vi "SteeringControl.vi"(0 "Position (Counts)":i32, 5 "Cluster":cluster{dbl, dbl, dbl}, 7 "P gain":dbl, 9 "I gain":dbl, 11 "D gain":dbl) -> (4 "Duty cycle":dbl, 6 "C out":dbl)   [LabVIEW 2019]
uses:
  usr/local/lib/libbalancing.so
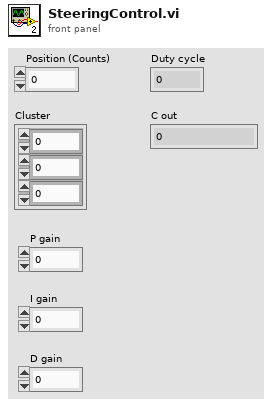
[diagram p1: front panel]
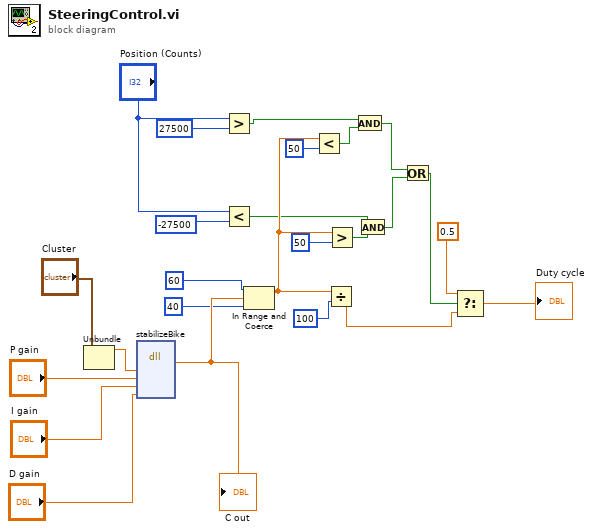
[diagram p0: block diagram]
diagram:
  n1 = Unbundle("Cluster") -> (w4:dbl)  [unwired: 2 out]
  n2 = dll-call lib="usr/local/lib/libbalancing.so" fn="stabilizeBike"("rollRate"=w4, "Kp"="P gain", "Ki"="I gain", "Kd"="D gain") -> ("return type"=w7:dbl)  [unwired: 7 in, 2 out]
  "C out" <- w7
  n3 = Greater?(x="Position (Counts)", y=27500) -> (0:w25:bool)
  n4 = Less?(x="Position (Counts)", y=-27500) -> (x < y?=w12:bool)
  n5 = In Range and Coerce(upper limit=60, x=w7, lower limit=40) -> (coerced(x)=w16:dbl)  [unwired: 1 out]
  n6 = Less?(x=w16, y=50) -> (x < y?=w15:bool)
  n7 = Divide(x=w16, y=100) -> (x/y=w21:dbl)
  n8 = Greater?(x=w16, y=50) -> (0:w13:bool)
  n9 = And(x=w25, y=w15) -> (x .and. y?=w18:bool)
  n10 = And(x=w12, y=w13) -> (x .and. y?=w19:bool)
  n11 = Or(x=w18, y=w19) -> (x .or. y?=w20:bool)
  n12 = Select(t=0.5, s=w20, f=w21) -> (s? t:f=→"Duty cycle":dbl)
